vi "PID Get Advanced Error (DBL).vi"(6 "setpoint range":cluster{"setpoint high":dbl, "setpoint low":dbl}, 7 "linearity":dbl, 8 "Gamma":dbl format="%#.7g", 9 "process variable":dbl, 10 "beta":dbl, 11 "setpoint":dbl) -> (0 "error with gamma":dbl, 1 "non-linear integral action":dbl, 2 "error with beta":dbl, 3 "error":dbl)   [LabVIEW 2020, in "NI_PID_pid.lvlib"]
uses:
  NI_PID_pid.lvlib
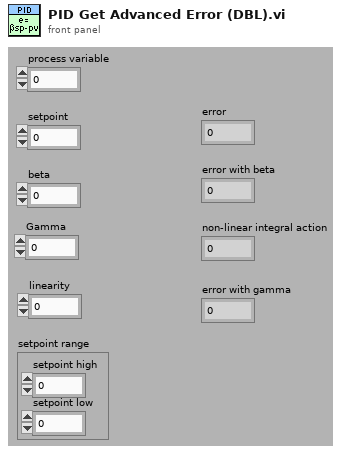
[diagram p1: front panel]
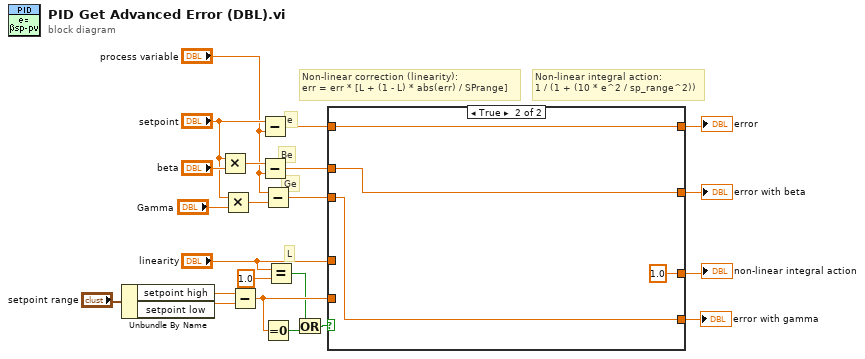
[diagram p0: block diagram]
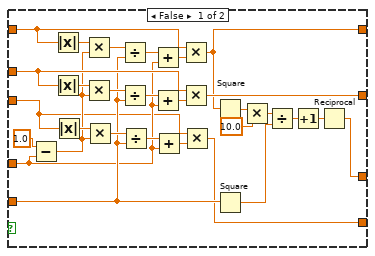
[diagram p2: hidden frame]
diagram:
  # "Ge"
  # "Non-linear correction (linearity):\nerr = err * [L + (1 - L) * abs(err) / SPrange]"
  # "Non-linear integral action:\n1 / (1 + (10 * e^2 / sp_range^2))"
  # "Be"
  # "e"
  # "L"
  n1 = Unbundle By Name("setpoint range") -> ("setpoint high"=w15:dbl, "setpoint low"=w14:dbl)
  n2 = Multiply(x="setpoint", y="beta") -> (x*y=w19:dbl)
  n3 = Multiply(x="setpoint", y="Gamma") -> (x*y=w6:dbl)
  n4 = Subtract(x=w15, y=w14) -> (x-y=w22:dbl)
  n5 = Subtract(x="setpoint", y="process variable") -> (x-y=w20:dbl)
  n6 = Subtract(x=w19, y="process variable") -> (x-y=w21:dbl)
  n7 = Subtract(x="process variable", y=w6) -> (x-y=w2:dbl)
  n8 = Equal To 0?(x=w22) -> (x = 0?=w7:bool)
  n9 = Equal?(x="linearity", y=1.0) -> (x = y?=w8:bool)
  n10 = Or(x=w8, y=w7) -> (x .or. y?=w9:bool)
  n11 = case shown="True" w9 {
    tunnel: [w38 1.0 ("t")] -> w16
    tunnel: w20 -> [w42 w54]
    tunnel: w21 -> [w43 w53]
    tunnel: [w36 w54] -> w17
    tunnel: [w41 w53] -> w18
    tunnel: w22 -> [w26 _]
    tunnel: "linearity" -> [w25 _]
    tunnel: w2 -> [w24 w52]
    tunnel: [w23 w52] -> w1
    frame False {
      n12 = Subtract(x=1.0, y=w25) -> (x-y=w27:dbl)
      n13 = Absolute Value(x=w42) -> (abs(x)=w51:dbl)
      n14 = Absolute Value(x=w43) -> (abs(x)=w44:dbl)
      n15 = Absolute Value(x=w24) -> (abs(x)=w31:dbl)
      n16 = Multiply(x=w51, y=w27) -> (x*y=w50:dbl)
      n17 = Multiply(x=w44, y=w27) -> (x*y=w45:dbl)
      n18 = Multiply(x=w31, y=w27) -> (x*y=w30:dbl)
      n19 = Divide(x=w50, y=w26) -> (x/y=w49:dbl)
      n20 = Divide(x=w45, y=w26) -> (x/y=w46:dbl)
      n21 = Divide(x=w30, y=w26) -> (x/y=w29:dbl)
      n22 = Add(x=w49, y=w25) -> (x+y=w48:dbl)
      n23 = Add(x=w46, y=w25) -> (x+y=w47:dbl)
      n24 = Add(x=w29, y=w25) -> (x+y=w28:dbl)
      n25 = Multiply(x=w42, y=w48) -> (x*y=w36:dbl)
      n26 = Multiply(x=w43, y=w47) -> (x*y=w41:dbl)
      n27 = Multiply(x=w24, y=w28) -> (x*y=w23:dbl)
      n28 = Square(x=w36) -> (x^2=w34:dbl)
      n29 = Square(x=w26) -> (x^2=w40:dbl)
      n30 = Multiply(x=w34, y=10.0) -> (x*y=w33:dbl)
      n31 = Divide(x=w33, y=w40) -> (x/y=w37:dbl)
      n32 = Increment(x=w37) -> (x+1=w39:dbl)
      n33 = Reciprocal(x=w39) -> (1/x=w38:dbl)
    }
    frame True {
    }
  }
  "error with beta" <- w18
  "error" <- w17
  "non-linear integral action" <- w16
  "error with gamma" <- w1
